vi "Polymorphic Add.vi"   [LabVIEW 2014]
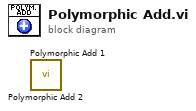
[diagram p0: block diagram]
diagram:
  n1 = call "Polymorphic Add 2.vi"() -> ()  [unwired: 10 in, 2 out]
  n2 = call "Polymorphic Add 1.vi"() -> ()  [unwired: 10 in, 2 out]
